vi "Gas_Setup.vi"() -> ()   [LabVIEW 2013]
uses:
  ADAM Controls/Ch_description_ADAM.ctl
  ADAM Controls/Module_type_ADAM.ctl
  ADAM Controls/Function_ADAM.ctl
  ADAM Controls/Channel_State.ctl
  ADAM Controls/Calib_type_ADAM.ctl
  ADAM Controls/Address.ctl
  ADAM Controls/Shut_Off_Valve.ctl
  ADAM Controls/Channel_names.ctl
  ADAM Controls/Update_scan_value.ctl
  Anemometry/Anemometry Sub Vis/Globals/Preference_global.vi
panel:
  out "Ch names":string[](array[string])
  in  "Select Plug Ins":bool
  in  "Source Info":string[][](table)
  in  "Trace Very Low":T1
  in  "Carrier 1 Very Low":T1
  in  "Carrier 1 Hi-Tec Range":u16(ring) items=["Very Low", "Low", "High"]
  in  "Trace Hi-Tec Range":u16(ring) items=["Very Low", "Low", "High"]
  in  "Carrier 1 High":T1
  in  "Carrier 1 Low":T1
  in  "Trace Low":T1
  in  "Trace High":T1
  in  "Release Orientation":u16(ring) items=["Vertical", "Horizontal 0 Deg", "Downwards", "External System Tests", "Horizontal", "Edit Strings"]
  in  "Source Type":u16(ring) items=["11mm downward facing", "1mm Annulus above tank wall with Internal 2mm Annulus floating roof at 50mm.", "23mm IDD=8mm", "2mm Annulus around a quarter of inside of tank wall", "2mm Annulus around inside of tank wall", "4 point source ID=8.5mm located 90 deg apart on 8cm Diameter", "8mm Annulus around inside of tank wall", "B2 D=6.8mm", "B204 Height 244mm ID 5.5mm", "B230 Height 152.4mm ID 8.5mm", "B30 Area", "B311 ID=11mm", "B331 ID=5.4mm", "B38_8mm_ID_passive", "B38_OD=3.1mm_ID=2mm", "B548 OD=13.8mm ID=3.5mm", "D=12mm", "D=13.6mm", "D=16mm (ID=12 mm)", "D=18mm", "D=20mm", "D=22.5mm", "D=3.4mm", "D=5mm (ground release)", "D=6mm (ID=4.2 mm)", "D=7.1mm", "D=9mm", "D=9mm  20mm long passive", "Dext = 8.5 mm", "Exit Port of Solenoid Valve", "H=25:W=100mm", "H=50", "ID=15 mm 90 deg bend copper tube", "ID=5.1mm OD=5.8mm (Ground release)", "ID=5.1mm OD=5.8mm (roof release)", "ID=5mm OD=5.8mm", "ID=8.5mm OD=10mm", "ID=9.5mm OD=12.5mm", "Line Source 100mm  1.07m width", "Line Source 25mm  1.3m long  perp to flow", "Line Source 25x1300", "Line Source 50mm  1.07m Wide", "Line source parallel to flow", "None", "ROSE 9mm at last grid", "SAV ID=3.5mm", "Sample tubes in source", "Single 5mm Stack", "Single 7.9 mm stack", "THORP  ID=5.1mm", "Twin 5mm Stacks", "Twin Passive Stacks ID=8mm OD=8.7mm", "UKAEA ID=1.7mm", "W=50mm", "Edit Strings"]
  in  "Current Release Temp":dbl format="%.2f"
  in  "Release Temperature":u16(ring) items=["Enter Value", "EnFlo_Tunnel:Job:Name", "GMU:Source:Type", "GMU:Release:Orientation", "EnFlo_Tunnel:Obstacle/:Building", "EnFlo_Tunnel:Vorticity:Generators", "EnFlo_Tunnel:Roughness:Height", "EnFlo_Tunnel:Side Wall:Separation", "GMU:Trace:Gas", "GMU:Carrier 1:Gas", "GMU:Carrier 2:Gas", "GMU:Carrier 1:Hi-Tec Range", "GMU:Trace:Hi-Tec Range", "EnFlo_Tunnel:Obstacle:Orientation", "GMU:Source:Density Ratio", "GMU:Carrier 1:Dem Volt", "GMU:Carrier 2:Dem Volt", "GMU:Trace:Dem Volt", "GMU:Carrier 1:Meas Volt", "GMU:Carrier 2:Meas Volt", "GMU:Trace:Meas Volt", "GMU:Carrier 1:Meas Q", "GMU:Carrier 2:Meas Q", "GMU:Trace:Meas Q", "GMU:Carrier 1:Meas M_dot", "GMU:Carrier 2:Meas M_dot", "GMU:Trace:Meas M_dot", "GMU:Remaining:Nitrogen", "GMU:Remaining:Helium", "GMU:Remaining:CO2", "GMU:Remaining:Krypton", "GMU:Remaining:Ethane", "GMU:Remaining:Propane", "GMU:Calibration:Gas 1", "GMU:Calibration:Gas 2", "GMU:Signal FID:Calib Gas", "GMU:Source:Dem Q", "GMU:Source:Meas Q", "GMU:Source:Meas M_dot", "GMU:Source:Meas Density", "GMU:Source:Meas Den Ratio", "GMU:Source:Dem Strength", "GMU:Source:Meas Strength", "GMU:Source:Est Time", "GMU:Detector:Meas Current", "GMU:Detector:Strength", "Froude:NPL:Atmos_Press", "EnFlo Lab:Hygrometry:Rel Humidity", "EnFlo Lab:Hygrometry:Dew Point temp", "EnFlo Lab:Hygrometry:Air Temp", "GMU:Test:Ethane trip", "EnFlo_Tunnel:Safety:GMU_Watchdog", "EnFlo_Tunnel:Speed:Dem Velocity", "EnFlo_Tunnel:Speed:Calib Tweak", "EnFlo_Tunnel:Speed:Dem Current", "EnFlo_Tunnel:Usonic Fixed:Velocity", "EnFlo_Tunnel:Usonic Fixed:Direction", "EnFlo_Tunnel:Prop Y+ve:Velocity", "EnFlo_Tunnel:Prop Y-ve:Velocity", "EnFlo_Tunnel:Shaft:rpm", "EnFlo_Tunnel:Reference:Velocity", "EnFlo_Tunnel:Hydrosonic:Integral", "EnFlo_Tunnel:Days Run at:2.5m/s", "Hydrosonic:Transducer:Setting", "EnFlo_Tunnel:Trav Origin:X Offset", "EnFlo_Tunnel:Trav Pos:X", "EnFlo_Tunnel:Trav Pos:Y", "EnFlo_Tunnel:Trav Pos:Z", "EnFlo Lab:labstrat1:Z=4.5m", "EnFlo Lab:labstrat1:Z=3.5m", "EnFlo Lab:labstrat1:Z=2.5m", "EnFlo Lab:labstrat1:Z=1.5m", "EnFlo Lab:labstrat1:Z=0.5m", "EnFlo Lab:labstrat1:Delta T", "EnFlo Lab:Desired:Air Temp", "EnFlo Lab:Heat:Extraction", "EnFlo Lab:labstrat1:Av Temp", "University:Outside:Temp", "EnFlo_Tunnel:Inlet Heater:Temp 1", "EnFlo_Tunnel:Inlet Heater:Temp 2", "EnFlo_Tunnel:Inlet Heater:Temp 3", "EnFlo_Tunnel:Inlet Heater:Temp 4", "EnFlo_Tunnel:Inlet Heater:Temp 5", "EnFlo_Tunnel:Inlet Heater:Temp 6", "EnFlo_Tunnel:Inlet Heater:Temp 7", "EnFlo_Tunnel:Inlet Heater:Temp 8", "EnFlo_Tunnel:Inlet Heater:Temp 9", "EnFlo_Tunnel:Inlet Heater:Temp 10", "EnFlo_Tunnel:Inlet Heater:Temp 11", "EnFlo_Tunnel:Inlet Heater:Temp 12", "EnFlo_Tunnel:Inlet Heater:Temp 13", "EnFlo_Tunnel:Inlet Heater:Temp 14", "EnFlo_Tunnel:Inlet Heater:Temp 15", "EnFlo_Tunnel:Inlet Heater:Av Temp", "EnFlo_Tunnel:Inlet Heater:Max Temp", "EnFlo_Tunnel:Heater:Enable", "EnFlo_Tunnel:floor near:1", "EnFlo_Tunnel:floor near:3", "EnFlo_Tunnel:floor near:5", "EnFlo_Tunnel:floor far:7", "EnFlo_Tunnel:floor near:7", "EnFlo_Tunnel:floor far:9", "EnFlo_Tunnel:floor near:10", "EnFlo_Tunnel:floor near:11", "EnFlo_Tunnel:floor far:11", "EnFlo_Tunnel:Exit Duct:Temp", "EnFlo_Tunnel:Parker X:Temp", "EnFlo_Tunnel:roof near:19", "EnFlo_Tunnel:roof far:19", "EnFlo_Tunnel:Fan Gearbox:Y+ Temp", "EnFlo_Tunnel:Fan Gearbox:Y- Temp", "B_Tunnel:Motor:Temp", "Uni:Chilled Water:Temp", "EnFlo_Tunnel:Chilled Water:Motor1 Temp", "EnFlo_Tunnel:Chilled Water:Motor2 Temp", "EnFlo_Tunnel:Chilled Water:Supply", "EnFlo_Tunnel:Chilled Water:Return", "EnFlo_Tunnel:Chilled Water:Dem Temp", "EnFlo_Tunnel:Chilled Water:Valve Dem Pos", "EnFlo_Tunnel:Chilled Water:Valve Dem Voltage", "A_Tunnel:Trav:1", "A_Tunnel:Speed:Dem Velocity", "A_Tunnel:Speed:Calib Tweak", "A_Tunnel:Speed:Dem Voltage", "A_Tunnel:Motor:Temp", "GMU:Source:Release Temp", "Complete:Scan:Period", "D_Tunnel:Motor:Temp", "Cluster Room:General:Temp", "Cluster Room:Temp:Warning", "D_Tunnel:Speed:Dem Velocity", "D_Tunnel:Speed:Calib Tweak", "D_Tunnel:Speed:Dem Voltage", "EnFlo Lab:Underfloor Tank:Temp", "Laser:Cooling water:Return Temp", "EnFlo_Tunnel:User:Name", "A_Tunnel:User:Name", "D_Tunnel:User:Name", "Paul_Hayden:User:Name", "Uni:Chilled Water:Temp Warning", "Frauke_Desktop:User:Name", "ADAM_Server:User:Name", "Calibration_Tunnel:User:Name", "EnFlo_Tunnel:Side near:10", "EnFlo_Tunnel:Side far:10", "EnFlo_Tunnel:Source_Pos:X", "EnFlo_Tunnel:Source_Pos:Y", "EnFlo_Tunnel:Source_Pos:Z", "EnFlo_Tunnel:Max_Surface:Temp", "EnFlo_Tunnel:Chiller_Pump:Enable", "A_Tunnel:Motor:Enable", "GMU:Source:Divertor Valve", "EnFlo_Tunnel:Tap_Water:Enable", "EnFlo_Tunnel:Cooling_Panel:Manifold_Temp", "EnFlo_Tunnel:Motor:Enable", "EnFlo_Tunnel:Lights:Enable", "EnFlo_Tunnel:FFID:Temp", "GMU:Gas:Enable", "GMU:Detector:Happy", "EnFlo_Tunnel:Gas Solenoid:Status", "EnFlo_Tunnel:Usonic Inlet Z=75:Velocity", "EnFlo_Tunnel:Usonic Inlet Z=75:Direction", "GMU:Source:Pressure", "EnFlo_Tunnel:Wind:Direction", "Status:of:PB_G4_2", "PB_G4_2:User:Name", "EnFlo Lab:Comp Air:Pressure", "EnFlo Lab:Leak_Detector:Happy", "Paul_Desk:User:Name", "EnFlo Lab:Comp Air:Warning", "EnFlo_Tunnel:Turbine_1:Dem_Volts", "Laser:Cooling_Pump:Enable", "LDA:System:Enable", "FFID:System:Enable", "EnFlo_Tunnel:Motor:Temp", "Laser:Cooling water:Temp Warning", "GMU:Trace:Open", "No Match::", "EnFlo_Tunnel:Chiller_Pump:Running", "EnFlo_Tunnel:Parker X:Warning Temp", "B_Tunnel:User:Name", "EnFlo_Tunnel:Heat_Ex_Water:Return Temp", "EnFlo_Tunnel:Exit Duct Top:Temp", "LDA:3 Phase:Power", "Hydrosonic:Seeder:Enable", "Sugar:Water:Temp", "Hydrosonic:Tank:Temp", "A_Tunnel:Turbine:Enable", "A_Tunnel:Turbine_1:Dem_Volts"]
  in  "Gas Remaining":string[][](table)
  in  "Signal FID Calib Gas":dbl format="%.2f"
  in  "Signal FID Calib Channel":u16(ring) items=["Input Value", "Channel 1", "Channel 2"]
  in  "Channel 2":dbl format="%.2f"
  in  "Channel 1":dbl format="%.2f"
  in  "Carrier 2 Gas":u16(ring) items=["Air", "Nitrogen", "Helium", "CO2", "Krypton", "None"]
  in  "Trace Gas":u16(ring) items=["Propane", "Ethane"]
  in  "Carrier 1 Gas":u16(ring) items=["Air", "Nitrogen", "Helium", "CO2", "Krypton", "None"]
  out "Numerical Values":dbl[](array[numeric]) format="%.9f"
  out "Ch Description Array":T2[](array[typedef]) {"Duty" format="%.0b"; "D" format="%#_5g"; "C" format="%#_5g"; "B" format="%#_5g"; "A" format="%#_5g"}
  out "dup reference":refnum<vi>
  in  "stop":bool
  in  "OK":bool
  # "Calibration Gas (ppm)"
  # "Very\nLow\nRange"
  # "High\nRange"
  # "Low\nRange"
  # "Low\nRange"
  # "Very\nLow\nRange"
  # "High\nRange"
  # "Dispersion Setup"
  # "To Source"
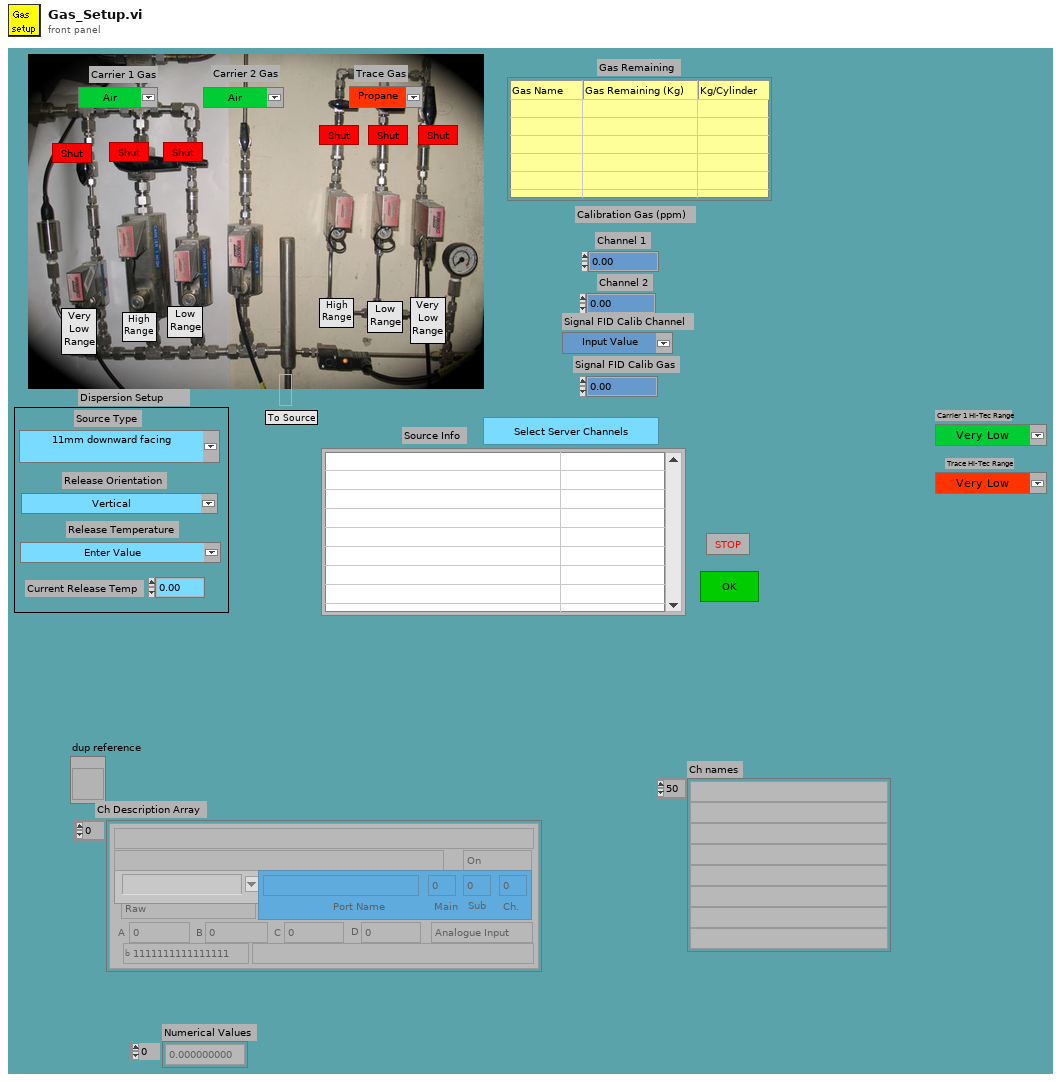
[diagram p1: front panel]
types:
  T1 = typedef "Shut_Off_Valve.ctl" = bool
  T2 = typedef "Ch_description_ADAM.ctl" = cluster{"Ch Name":string, "Type":T3, "Function":T4, "Ch State":T5, "Calibration type":T6, "A":dbl, "B":dbl, "C":dbl, "D":dbl, "Comments":string, "Address":T7, "String":string, "Duty":u16}
  T3 = typedef "Module_type_ADAM.ctl" = string
  T4 = typedef "Function_ADAM.ctl" = enum16{"Analogue Input", "Digital Input", "Event counter", "Event rate", "Analogue Output", "Digital Output", "Relay Output"}
  T5 = typedef "Channel_State.ctl" = enum16{"On", "Off", "Always On", "Always Off"}
  T6 = typedef "Calib_type_ADAM.ctl" = enum16{"Raw", "Bx + A", "Cx^2 + Bx + A", "Dx^3 + Cx^2 + Bx + A", "In Band", "Hi-Tec Q", "Hi-Tec M_dot", "Text"}
  T7 = typedef "Address.ctl" = cluster{"Main":i32, "Ch.":i32, "Sub":i32, "Port Name":string}
  T8 = typedef "Channel_names.ctl" = enum16{"Active Only", "Active + Off", "All Channels"}
  T9 = typedef "Update_scan_value.ctl" = cluster{"Channel Name":string, "New Value":dbl}
  T10 = enum16{"Zero or one", "One", "Zero or more", "One or more"}
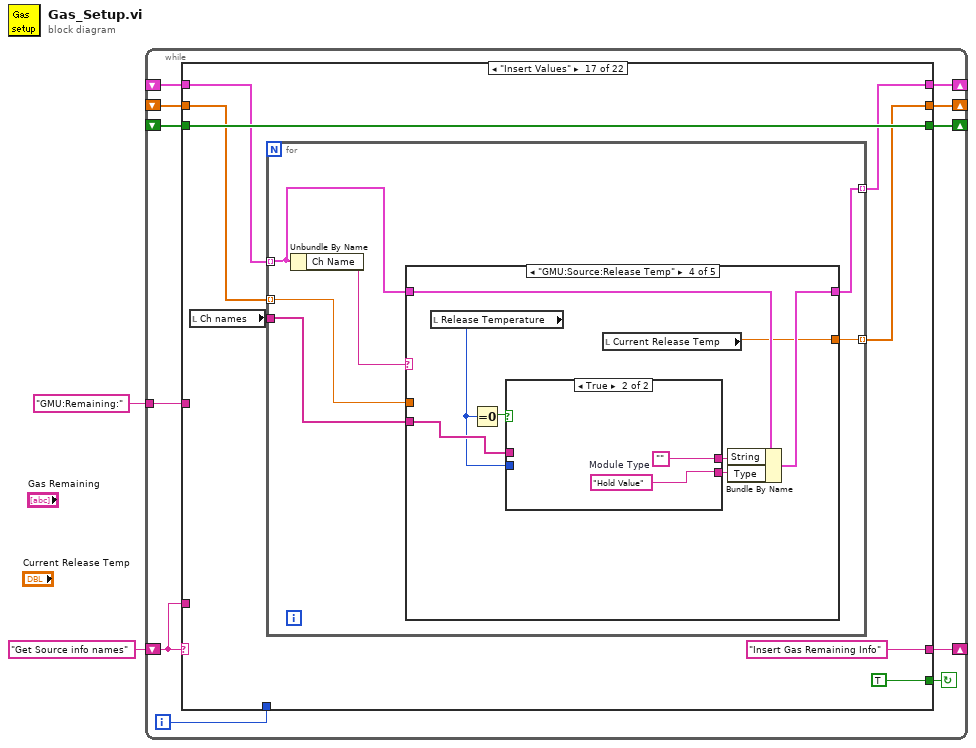
[diagram p0: block diagram]
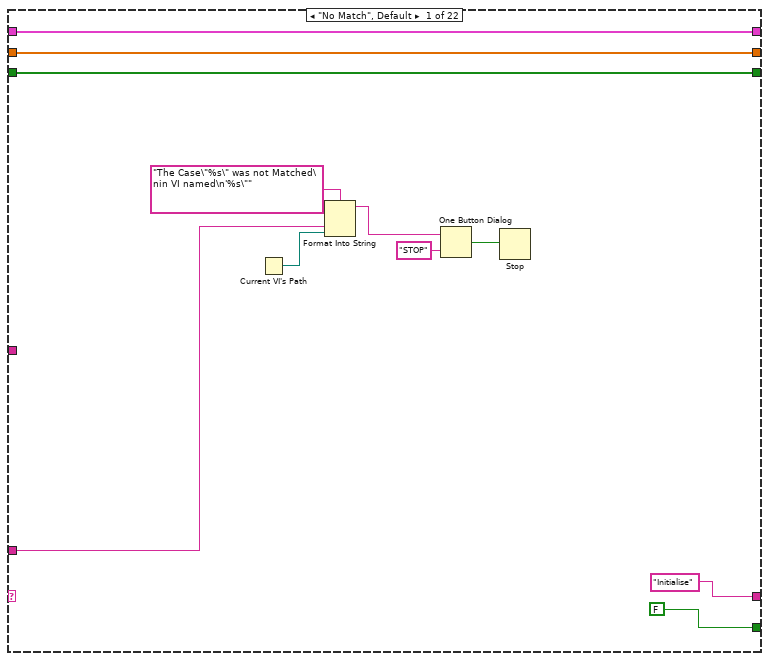
[diagram p2: hidden frame]
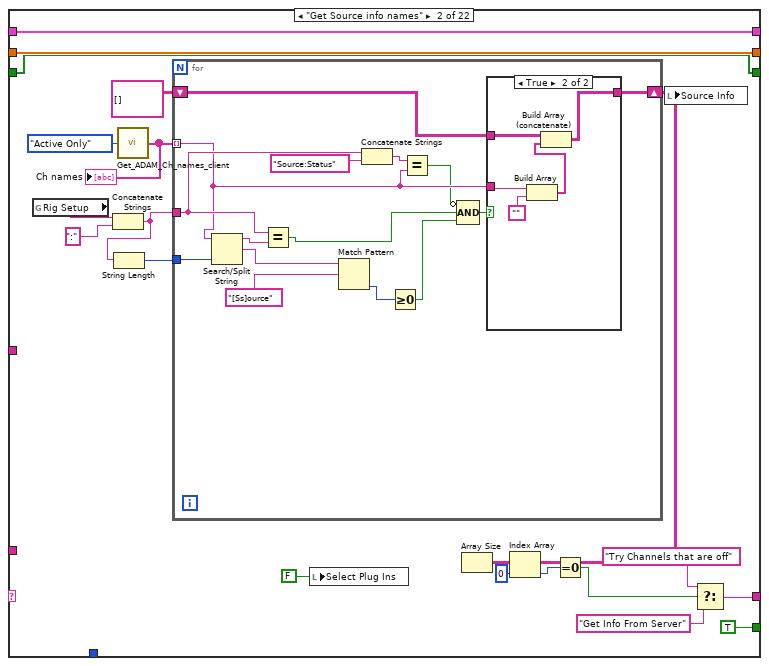
[diagram p3: hidden frame]
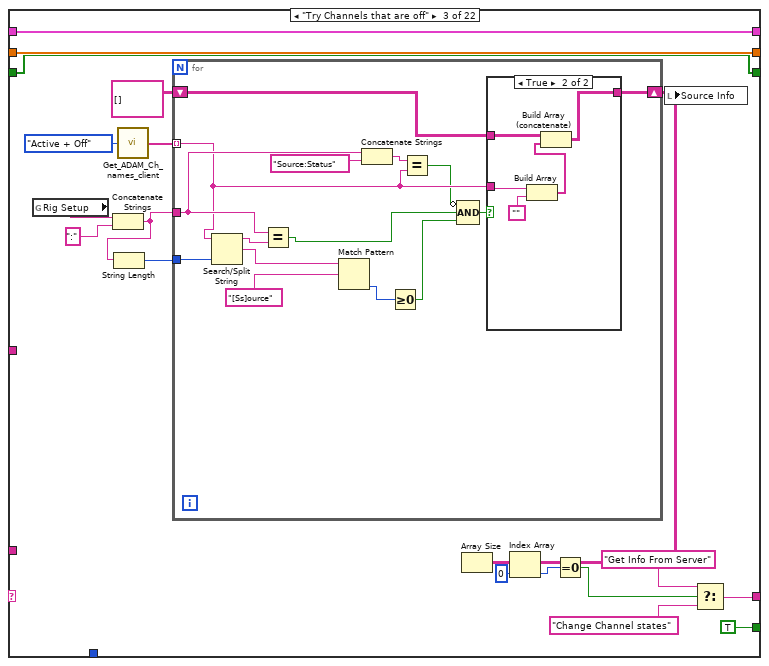
[diagram p5: hidden frame]
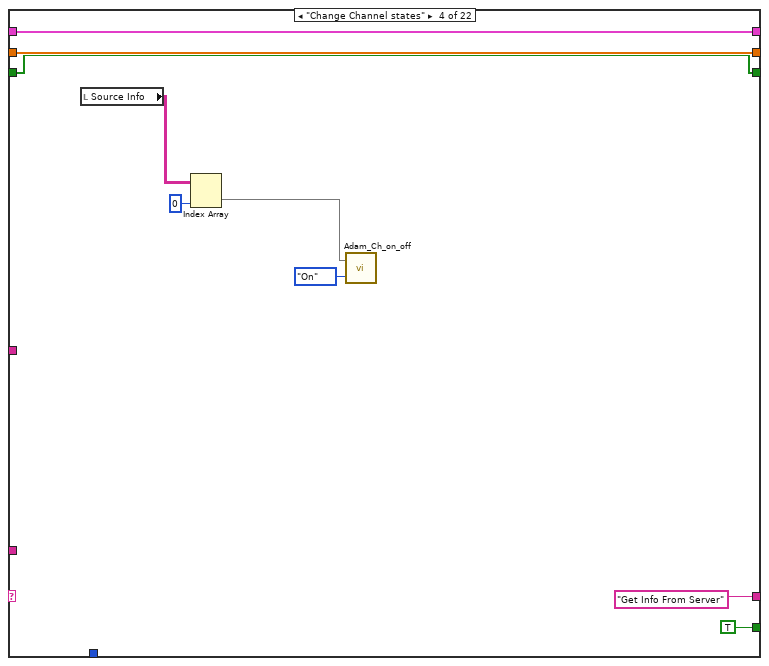
[diagram p7: hidden frame]
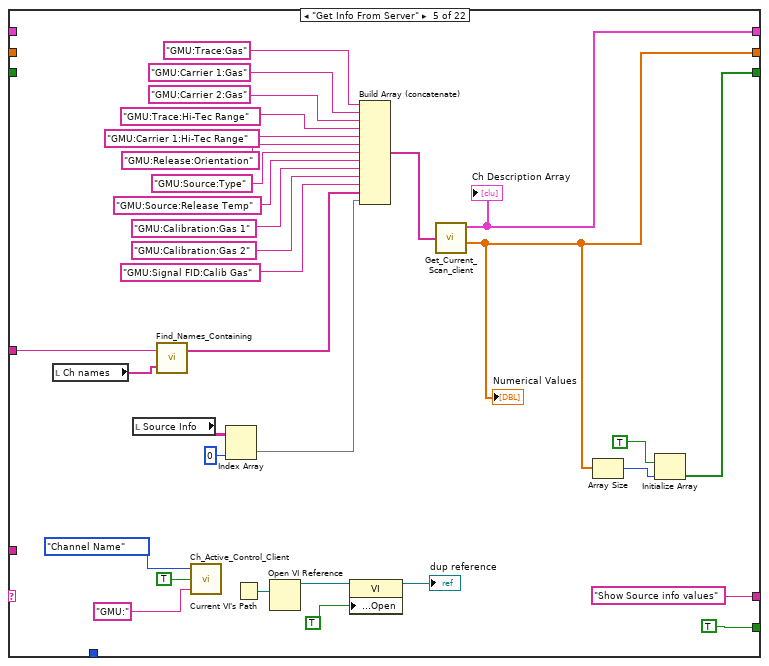
[diagram p8: hidden frame]
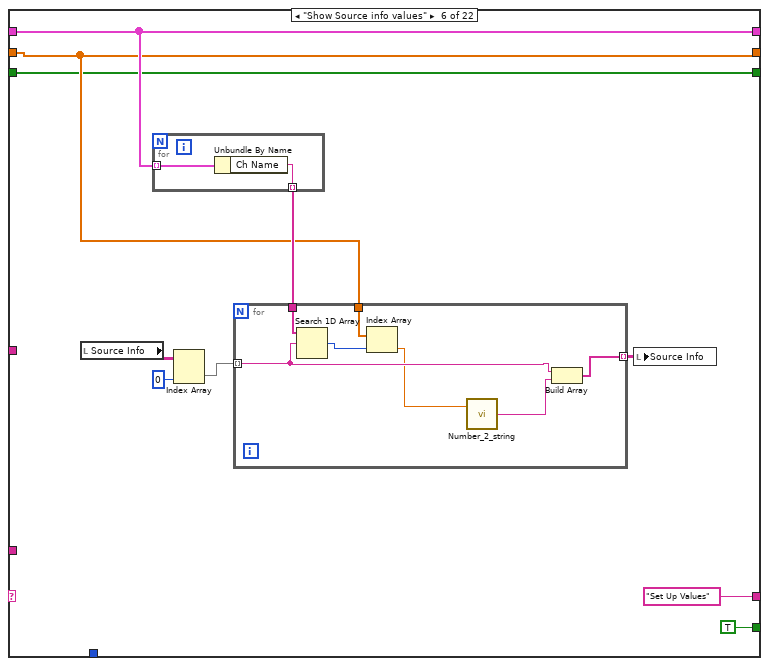
[diagram p9: hidden frame]
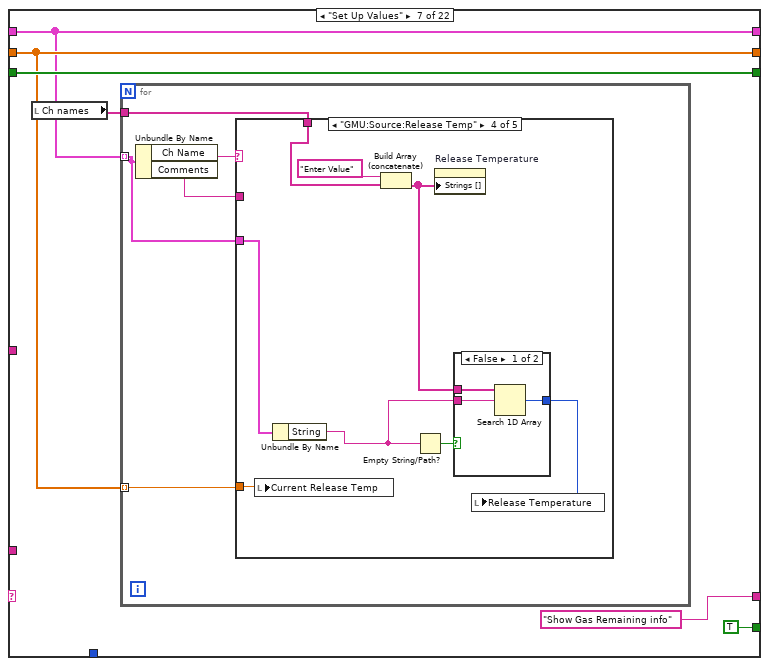
[diagram p10: hidden frame]
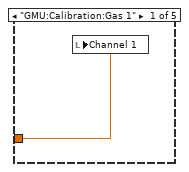
[diagram p11: hidden frame]
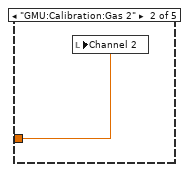
[diagram p12: hidden frame]
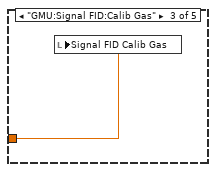
[diagram p13: hidden frame]
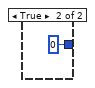
[diagram p14: hidden frame]
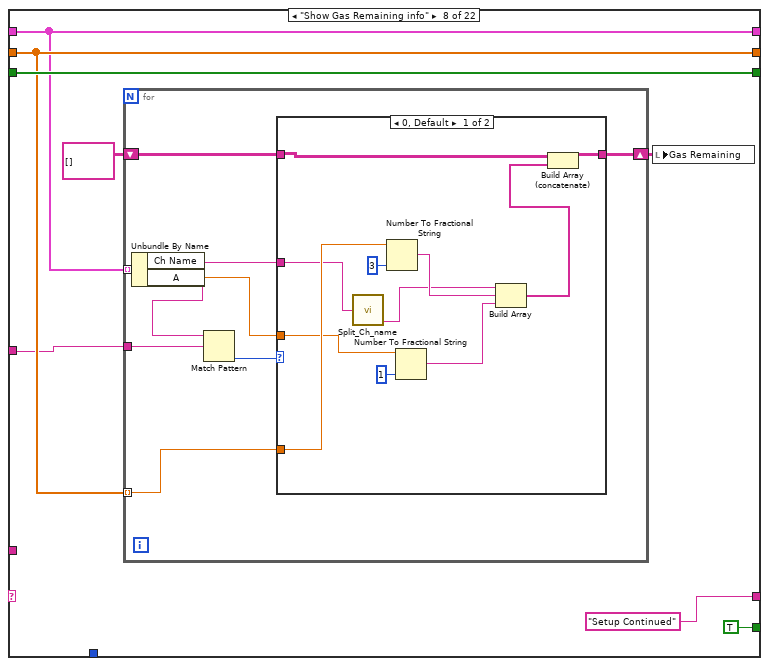
[diagram p16: hidden frame]
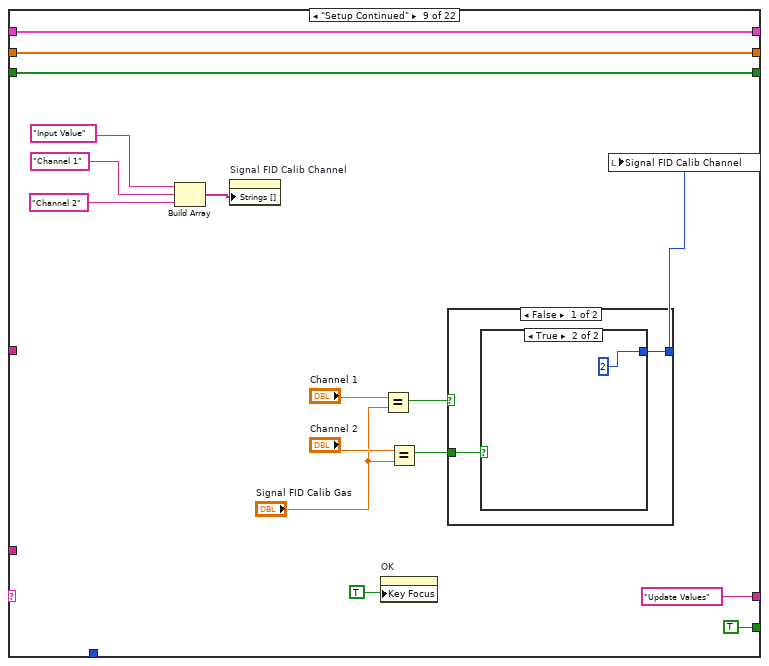
[diagram p18: hidden frame]
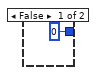
[diagram p19: hidden frame]
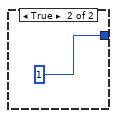
[diagram p20: hidden frame]
diagram:
  n1 = while {
    shift-left: _ -> [w5]
    shift-right: [w6] -> _
    shift-left: _ -> [w7]
    shift-right: [w9] -> _
    shift-left: _ -> [w8]
    shift-right: [w10] -> _
    shift-left: "Get Source info names" ("t") -> [w11]
    shift-right: [w12] -> _
    tunnel: "GMU:Remaining:" -> [w3]
    i -> [w4]
    stop <- w13 continue-if-true
    n2 = case shown="\"Insert Values\"" w11 {
      tunnel: [FALSE TRUE ("T button?") TRUE ("T button?") TRUE ("T button?") TRUE TRUE ("T button?") TRUE ("T button?") TRUE ("T button?") TRUE ("T button?") TRUE ("T button?") TRUE ("T button?") TRUE ("T button?") TRUE ("T button?") TRUE ("T button?") TRUE ("T button?") TRUE ("T button?") TRUE ("T button?") TRUE ("T button?") TRUE ("T button?") TRUE ("T button?") TRUE ("T button?") FALSE ("T button?")] -> w13
      tunnel: ["Initialise" w26 w68 "Get Info From Server" "Show Source info values" "Set Up Values" "Show Gas Remaining info" "Setup Continued" "Update Values" "Slow FID Calib Gas" w324 "Update Release Temperature" "Sort out Valve Logic" "Hi Tec Ranges" "Continue looping?" w468 "Insert Gas Remaining Info" "Insert Source info values" "Update Server" w566 "Get Source info names" ("t") "End"] -> w12
      tunnel: w11 -> [w19 _ _ _ _ _ _ _ _ _ _ _ _ _ _ _ _ _ _ _ _ _]
      tunnel: [w16 w40 w80 w114 w139 w155 w167 w195 w235 w246 w329 w347 w377 w394 w452 w474 w476 w515 w547 w575 w631 w682] -> w10
      tunnel: [w15 w39 w79 w113 w125 w154 w168 w196 w234 w244 w328 w346 w376 w393 w451 w473 w479 w521 w549 w574 w630 w681] -> w9
      tunnel: w8 -> [w16 w40 w80 w114 _ w155 w167 w195 w235 w247 w329 w347 w377 w394 w452 w474 w477 w515 w547 w575 w631 w682]
      tunnel: w7 -> [w15 w39 w79 w113 _ w154 w168 w196 w234 w245 w328 w346 w376 w393 w451 w473 w478 w520 w550 w574 w630 w681]
      tunnel: [w14 w38 w78 w112 w124 w153 w170 w198 w232 w241 w322 w344 w374 w391 w449 w467 w481 w523 w546 w573 w629 w674] -> w6
      tunnel: w5 -> [w14 w38 w78 w112 _ w153 w170 w198 w232 w242 w322 w344 w374 w391 w449 w467 w481 w523 w546 w573 w629 w674]
      tunnel: w4 -> [_ _ _ _ _ _ _ _ _ _ w321 _ _ _ _ _ _ _ _ _ _ _]
      tunnel: w3 -> [_ _ _ _ w122 _ _ w194 _ _ _ _ _ _ _ _ _ w514 _ _ _ _]
      frame "No Match", Default {
        n3 = Current VI's Path() -> (path=w18:path)
        n4 = Format Into String(format string="The Case\"%s\" was not Matched\nin VI named\n'%s\"" ("Format String"), w19, w18) -> (resulting string=w22:string)  [unwired: 2 in, 1 out]
        n5 = One Button Dialog(message=w22, button name ("OK")="STOP") -> (true=w20:bool)
        n6 = Stop(stop? (T)=w20) -> ()
      }
      frame "Get Source info names" {
        n7 = global read "Preference_global.vi" "Rig Setup"() -> (w44:string)
        n8 = Concatenate Strings(w44, ":" ("string")) -> (w41:string)
        n9 = String Length(string=w41) -> (length=w42:i32)
        n10 = call "Get_ADAM_Ch_names_client.vi"("Channel names set"=Channel_names."Active Only") -> ("Ch names"=w35:string[])
        "Ch names" <- w35
        n11 = for {
          tunnel: w42 -> [w59]
          tunnel: w35 -> [w49] mode=indexing
          tunnel: w41 -> [w51]
          shift-right: [w53] -> w33
          shift-left: string[][] [] -> [w54]
          n12 = Search/Split String(string=w49, offset (0)=w59) -> (substring before match=w58:string, match + rest of string=w57:string)  [unwired: 2 out]
          n13 = Equal?(x=w51, y=w58) -> (x = y?=w47:bool)
          n14 = Match Pattern(string=w57, regular expression="[Ss]ource") -> (offset past match=w55:i32)  [unwired: 4 out]
          n15 = Concatenate Strings(w51, "Source:Status") -> (w50:string)
          n16 = Greater Or Equal To 0?(x=w55) -> (x >= 0?=w48:bool)
          n17 = Equal?(x=w50, y=w49) -> (x = y?=w46:bool)
          n18 = Compound Arithmetic op=AND(invert w46, w47, w48) -> (w45:bool)
          n19 = case shown="True" w45 {
            tunnel: w54 -> [w60 w65]
            tunnel: w49 -> [_ w63]
            tunnel: [w60 w64] -> w53
            frame False {
            }
            frame True {
              n20 = Build Array(w63, "") -> (w61:string[])
              n21 = Build Array (concatenate)(w65, w61) -> (w64:string[][])
            }
          }
        }
        n22 = local write "Select Plug Ins"(FALSE ("Select Plug Ins")) -> ()
        n23 = Array Size(array=w33) -> (size(s)=w32:i32[])
        n24 = Index Array(array=w32, index=0) -> (element=w30:i32)
        n25 = Equal To 0?(x=w30) -> (x = 0?=w28:bool)
        n26 = local write "Source Info"(w33) -> ()
        n27 = Select(t="Try Channels that are off", s=w28, f="Get Info From Server") -> (s? t:f=w26:string)
      }
      frame "Try Channels that are off" {
        n28 = global read "Preference_global.vi" "Rig Setup"() -> (w84:string)
        n29 = Concatenate Strings(w84, ":" ("string")) -> (w81:string)
        n30 = String Length(string=w81) -> (length=w82:i32)
        n31 = call "Get_ADAM_Ch_names_client.vi"("Channel names set"=Channel_names."Active + Off") -> ("Ch names"=w75:string[])
        n32 = for {
          tunnel: w82 -> [w99]
          tunnel: w75 -> [w89] mode=indexing
          tunnel: w81 -> [w91]
          shift-right: [w93] -> w74
          shift-left: string[][] [] -> [w94]
          n33 = Search/Split String(string=w89, offset (0)=w99) -> (substring before match=w98:string, match + rest of string=w97:string)  [unwired: 2 out]
          n34 = Equal?(x=w91, y=w98) -> (x = y?=w87:bool)
          n35 = Match Pattern(string=w97, regular expression="[Ss]ource") -> (offset past match=w95:i32)  [unwired: 4 out]
          n36 = Concatenate Strings(w91, "Source:Status") -> (w90:string)
          n37 = Greater Or Equal To 0?(x=w95) -> (x >= 0?=w88:bool)
          n38 = Equal?(x=w90, y=w89) -> (x = y?=w86:bool)
          n39 = Compound Arithmetic op=AND(invert w86, w87, w88) -> (w85:bool)
          n40 = case shown="True" w85 {
            tunnel: w94 -> [w100 w105]
            tunnel: w89 -> [_ w103]
            tunnel: [w100 w104] -> w93
            frame False {
            }
            frame True {
              n41 = Build Array(w103, "") -> (w101:string[])
              n42 = Build Array (concatenate)(w105, w101) -> (w104:string[][])
            }
          }
        }
        n43 = Array Size(array=w74) -> (size(s)=w73:i32[])
        n44 = Index Array(array=w73, index=0) -> (element=w71:i32)
        n45 = Equal To 0?(x=w71) -> (x = 0?=w69:bool)
        n46 = local write "Source Info"(w74) -> ()
        n47 = Select(t="Get Info From Server", s=w69, f="Change Channel states") -> (s? t:f=w68:string)
      }
      frame "Change Channel states" {
        n48 = local read "Source Info"() -> (w109:string[][])
        n49 = Index Array(array=w109, index (col)=0 ("disabled index (col)")) -> (element=w107:string[])  [unwired: 1 in]
        n50 = call "Adam_Ch_on_off.vi"("Ch State"=Channel_State."On", "ADAM Ch Names"=w107) -> ()  [unwired: 1 out]
      }
      frame "Get Info From Server" {
        n51 = local read "Ch names"() -> (w115:string[])
        n52 = local read "Source Info"() -> (w118:string[][])
        n53 = call "Find_Names_Containing.vi"("Ch names"=w115, "String to match"=w122) -> ("Matched Names"=w123:string[])  [unwired: 1 out]
        n54 = call "Ch_Active_Control_Client.vi"("Match"="GMU:", "Activate Channels?"=TRUE, "Control on"=enum16{"Channel Name", "Main Address"}."Channel Name") -> ()  [unwired: 2 out]
        n55 = Index Array(array=w118, index (col)=0 ("disabled index (col)")) -> (element=w116:string[])  [unwired: 1 in]
        n56 = Current VI's Path() -> (path=w141:path)
        n57 = Open VI Reference(vi path=w141) -> (vi reference=w142:refnum<vi>)  [unwired: 1 in, 5 out]
        n58 = property class="VI"(reference=w142, "Front Panel Window:Open"=TRUE) -> (reference out=→"dup reference":refnum<vi>)  [unwired: 1 in, 1 out]
        n59 = Build Array (concatenate)("GMU:Trace:Gas", "GMU:Carrier 1:Gas", "GMU:Carrier 2:Gas", "GMU:Trace:Hi-Tec Range", "GMU:Carrier 1:Hi-Tec Range", "GMU:Release:Orientation", "GMU:Source:Type", "GMU:Source:Release Temp", "GMU:Calibration:Gas 1", "GMU:Calibration:Gas 2", "GMU:Signal FID:Calib Gas", w123, w116) -> (w144:string[])
        n60 = call "Get_Current_Scan_client.vi"("ADAM Ch Names"=w144) -> ("Ch Description Array"=w139:T2[], "Numerical Values"=w125:dbl[])  [unwired: 2 out]
        "Ch Description Array" <- w139
        "Numerical Values" <- w125
        n61 = Array Size(array=w125) -> (size(s)=w127:i32)
        n62 = Initialize Array(TRUE, w127) -> (w124:bool[])
      }
      frame "Show Source info values" {
        n63 = local read "Source Info"() -> (w149:string[][])
        n64 = for {
          tunnel: w155 -> [w165] mode=indexing
          tunnel: [w164] -> w156 mode=indexing
          n65 = Unbundle By Name(w165) -> ("Ch Name"=w164:string)
        }
        n66 = Index Array(array=w149, index (col)=0 ("disabled index (col)")) -> (element=w147:string[])  [unwired: 1 in]
        n67 = for {
          tunnel: w156 -> [w163]
          tunnel: w147 -> [w160] mode=indexing
          tunnel: w154 -> [w161]
          tunnel: [w157] -> w152 mode=indexing
          n68 = Search 1D Array(1D array=w163, element=w160) -> (index of element=w162:i32)  [unwired: 1 out]
          n69 = Index Array(array=w161, index=w162) -> (element=w159:dbl)
          n70 = call "Number_2_string.vi"("number"=w159) -> ("String"=w158:string)  [unwired: 1 in]
          n71 = Build Array(w160, w158) -> (w157:string[])
        }
        n72 = local write "Source Info"(w152) -> ()
      }
      frame "Set Up Values" {
        n73 = local read "Ch names"() -> (w166:string[])
        n74 = for {
          tunnel: w168 -> [w172] mode=indexing
          tunnel: w167 -> [w174] mode=indexing
          tunnel: w166 -> [w173]
          n75 = Unbundle By Name(w174) -> ("Ch Name"=w176:string, "Comments"=w175:string)
          n76 = case shown="\"GMU:Source:Release Temp\"" w176 {
            tunnel: w172 -> [w177 w178 w179 w183 _]
            tunnel: w175 -> [_ _ _ _ _]
            tunnel: w174 -> [_ _ _ w187 _]
            tunnel: w173 -> [_ _ _ w181 _]
            frame "GMU:Calibration:Gas 1" {
              n77 = local write "Channel 1"(w177) -> ()
            }
            frame "GMU:Calibration:Gas 2" {
              n78 = local write "Channel 2"(w178) -> ()
            }
            frame "GMU:Signal FID:Calib Gas" {
              n79 = local write "Signal FID Calib Gas"(w179) -> ()
            }
            frame "GMU:Source:Release Temp" {
              n80 = local write "Current Release Temp"(w183) -> ()
              n81 = Unbundle By Name(w187) -> ("String"=w185:string)
              n82 = Build Array (concatenate)("Enter Value", w181) -> (w180:string[])
              n83 = Empty String/Path?(string/path=w185) -> (empty?=w186:bool)
              n84 = property on="Release Temperature" class="Ring (strict)"("Strings []"=w180) -> ()  [unwired: 2 in, 2 out]
              n85 = case shown="False" w186 {
                tunnel: w180 -> [w190 _]
                tunnel: w185 -> [w189 _]
                tunnel: [w188 0 ("index of element")] -> w184
                frame False {
                  n86 = Search 1D Array(1D array=w190, element=w189) -> (index of element=w188:i32)  [unwired: 1 out]
                }
                frame True {
                }
              }
              n87 = local write "Release Temperature"(w184) -> ()
            }
            frame "No Match", Default {
            }
          }
        }
      }
      frame "Show Gas Remaining info" {
        n88 = for {
          tunnel: w196 -> [w202] mode=indexing
          tunnel: w195 -> [w207] mode=indexing
          tunnel: w194 -> [w206]
          shift-right: [w203] -> w192
          shift-left: string[][] [] -> [w204]
          n89 = Unbundle By Name(w207) -> ("Ch Name"=w200:string, "A"=w201:dbl)
          n90 = Match Pattern(string=w200, regular expression=w206) -> (offset past match=w205:i32)  [unwired: 4 out]
          n91 = case shown="0, Default" w205 {
            tunnel: w204 -> [w209 w219]
            tunnel: [w208 w219] -> w203
            tunnel: w202 -> [w213 _]
            tunnel: w201 -> [w212 _]
            tunnel: w200 -> [w211 _]
            frame 0, Default {
              n92 = call "Split_Ch_name.vi"("Ch name"=w211) -> ("Low level"=w215:string)  [unwired: 2 out]
              n93 = Number To Fractional String(number=w213, precision (6)=i16 3) -> (F-format string=w218:string)  [unwired: 2 out]
              n94 = Number To Fractional String(number=w212, precision (6)=i16 1) -> (F-format string=w216:string)  [unwired: 2 out]
              n95 = Build Array(w215, w218, w216) -> (w210:string[])
              n96 = Build Array (concatenate)(w209, w210) -> (w208:string[][])
            }
            frame -1 {
            }
          }
        }
        n97 = local write "Gas Remaining"(w192) -> ()
      }
      frame "Setup Continued" {
        n98 = Build Array("Input Value", "Channel 1", "Channel 2") -> (w226:string[])
        n99 = property on="Signal FID Calib Channel" class="Ring (strict)"("Strings []"=w226) -> ()  [unwired: 2 in, 2 out]
        n100 = property on="OK" class="Bool"("Key Focus"=TRUE ("Write Attribute")) -> ()  [unwired: 2 in, 2 out]
        n101 = Equal?(x="Channel 1", y="Signal FID Calib Gas") -> (x = y?=w225:bool)
        n102 = Equal?(x="Channel 2", y="Signal FID Calib Gas") -> (x = y?=w224:bool)
        n103 = case shown="False" w225 {
          tunnel: [w236 1] -> w220
          tunnel: w224 -> [w237 _]
          frame False {
            n104 = case shown="True" w237 {
              tunnel: [0 2] -> w236
              frame False {
              }
              frame True {
              }
            }
          }
          frame True {
          }
        }
        n105 = local write "Signal FID Calib Channel"(w220) -> ()
      }
      frame "Update Values" {
        n106 = for {
          tunnel: w247 -> [w254] mode=indexing
          tunnel: [w253] -> w246 mode=indexing
          tunnel: w245 -> [w252] mode=indexing
          tunnel: [w251] -> w244 mode=indexing
          tunnel: w242 -> [w250] mode=indexing
          tunnel: [w249] -> w241 mode=indexing
          n107 = Unbundle By Name(w254) -> ("Calibration type"=w257:T6, "String"=w256:string, "Ch Name"=w255:string)
          n108 = case shown="\"Text\"" w257 {
            tunnel: w256 -> [_ w278]
            tunnel: w255 -> [_ w268]
            tunnel: w254 -> [w260 w272]
            tunnel: [w260 w271] -> w253
            tunnel: w252 -> [w259 w270]
            tunnel: [w259 w269] -> w251
            tunnel: w250 -> [w258 w267]
            tunnel: [w258 w261] -> w249
            frame "Raw", Default {
            }
            frame "Text" {
              n109 = call "Get_array_values_fr_String.vi"("String Value"=w278) -> ("String array"=w265:string[])  [unwired: 1 out]
              n110 = To Unsigned Word Integer(number=w270) -> (unsigned 16bit integer=w276:u16)
              n111 = Build Array (concatenate)(w265, "Edit Strings") -> (w264:string[])
              n112 = Array Size(array=w265) -> (size(s)=w277:i32)
              n113 = case shown="\"GMU:Carrier 1:Hi-Tec Range\"" w268 {
                tunnel: [w285 w289 w294 w299 w303 w307 w312 w317] -> w262
                tunnel: w265 -> [_ w287 w291 w297 _ _ _ _]
                tunnel: w276 -> [w285 w290 w295 w300 w304 w308 w313 w318]
                tunnel: w267 -> [_ w288 w293 w298 w302 w306 w311 w316]
                tunnel: w264 -> [_ _ _ _ _ _ w310 w315]
                frame "No match", Default {
                }
                frame "GMU:Trace:Gas" {
                  n114 = property on="Trace Gas" class="Ring (strict)"("Strings []"=w287) -> ()  [unwired: 2 in, 2 out]
                  n115 = Select(t=w290, s=w288, f="Trace Gas") -> (s? t:f=w289:u16)
                  n116 = local write "Trace Gas"(w289) -> ()
                }
                frame "GMU:Carrier 1:Gas" {
                  n117 = property on="Carrier 1 Gas" class="Ring (strict)"("Strings []"=w291) -> ()  [unwired: 2 in, 2 out]
                  n118 = Select(t=w295, s=w293, f="Carrier 1 Gas") -> (s? t:f=w294:u16)
                  n119 = local write "Carrier 1 Gas"(w294) -> ()
                }
                frame "GMU:Carrier 2:Gas" {
                  n120 = property on="Carrier 2 Gas" class="Ring (strict)"("Strings []"=w297) -> ()  [unwired: 2 in, 2 out]
                  n121 = Select(t=w300, s=w298, f="Carrier 2 Gas") -> (s? t:f=w299:u16)
                  n122 = local write "Carrier 2 Gas"(w299) -> ()
                }
                frame "GMU:Carrier 1:Hi-Tec Range" {
                  n123 = Select(t=w304, s=w302, f="Carrier 1 Hi-Tec Range") -> (s? t:f=w303:u16)
                  n124 = local write "Carrier 1 Hi-Tec Range"(w303) -> ()
                }
                frame "GMU:Trace:Hi-Tec Range" {
                  n125 = Select(t=w308, s=w306, f="Trace Hi-Tec Range") -> (s? t:f=w307:u16)
                  n126 = local write "Trace Hi-Tec Range"(w307) -> ()
                }
                frame "GMU:Source:Type" {
                  n127 = property on="Source Type" class="Ring (strict)"("Strings []"=w310) -> ()  [unwired: 2 in, 2 out]
                  n128 = Select(t=w313, s=w311, f="Source Type") -> (s? t:f=w312:u16)
                  n129 = local write "Source Type"(w312) -> ()
                }
                frame "GMU:Release:Orientation" {
                  n130 = property on="Release Orientation" class="Ring (strict)"("Strings []"=w315) -> ()  [unwired: 2 in, 2 out]
                  n131 = Select(t=w318, s=w316, f="Release Orientation") -> (s? t:f=w317:u16)
                  n132 = local write "Release Orientation"(w317) -> ()
                }
              }
              n133 = To Unsigned Word Integer(number=w277) -> (unsigned 16bit integer=w275:u16)
              n134 = Equal?(x=w275, y=w262) -> (x = y?=w261:bool)
              n135 = case shown="True" w261 {
                tunnel: w265 -> [w280 w284]
                tunnel: w268 -> [_ w283]
                tunnel: [w280 w282] -> w273
                tunnel: [w279 w281] -> w263
                tunnel: w262 -> [w279 _]
                frame False {
                }
                frame True {
                  n136 = call "Edit_String_Options_list.vi"("Channel Name"=w283, "String array"=w284) -> ("New Selection Index"=w281:i32, "String array Out"=w282:string[])
                }
              }
              n137 = call "Put_Array_into_String.vi"("String array"=w273) -> ("String Value"=w274:string)
              n138 = Bundle By Name(cluster=w272, "String"=w274) -> (w271:T2)
              n139 = To Double Precision Float(number=w263) -> (double precision float=w269:dbl)
            }
          }
        }
      }
      frame "Slow FID Calib Gas" {
        n140 = Less?(x=w321, y=10) -> (x < y?=w319:bool)
        n141 = case shown="1, Default" "Signal FID Calib Channel" {
          tunnel: "Signal FID Calib Channel" -> [_ w331]
          frame 0 {
          }
          frame 1, Default {
            n142 = case shown="2" w331 {
              tunnel: [0.0 w333 w334] -> w330
              frame 0, Default {
              }
              frame 1 {
                n143 = local read "Channel 1"() -> (w333:dbl)
              }
              frame 2 {
                n144 = local read "Channel 2"() -> (w334:dbl)
              }
            }
            n145 = local write "Signal FID Calib Gas"(w330) -> ()
          }
        }
        n146 = Select(t="Initialise Hi tec selection", s=w319, f="Update Release Temperature") -> (s? t:f=w324:string)
      }
      frame "Initialise Hi tec selection" {
        n147 = local read "Carrier 1 Hi-Tec Range"() -> (w342:u16)
        n148 = local read "Trace Hi-Tec Range"() -> (w338:u16)
        n149 = case shown="2" w342 {
          tunnel: [FALSE FALSE TRUE] -> w341
          tunnel: [FALSE TRUE FALSE] -> w340
          tunnel: [TRUE FALSE FALSE] -> w339
          frame 0, Default {
          }
          frame 1 {
          }
          frame 2 {
          }
        }
        n150 = case shown="0, Default" w338 {
          tunnel: [FALSE FALSE TRUE] -> w335
          tunnel: [FALSE TRUE FALSE] -> w336
          tunnel: [TRUE FALSE FALSE] -> w337
          frame 0, Default {
          }
          frame 1 {
          }
          frame 2 {
          }
        }
        n151 = local write "Carrier 1 Very Low"(w339) -> ()
        n152 = local write "Carrier 1 High"(w341) -> ()
        n153 = local write "Carrier 1 Low"(w340) -> ()
        n154 = local write "Trace Very Low"(w337) -> ()
        n155 = local write "Trace Low"(w336) -> ()
        n156 = local write "Trace High"(w335) -> ()
      }
      frame "Update Release Temperature" {
        n157 = while {
          tunnel: [w380] -> w371
          shift-left: _ -> [w380]
          shift-right: [w381] -> w372
          stop <- FALSE continue-if-true
          n158 = Get Date/Time In Seconds() -> (seconds since 1Jan1904=w378:timestamp)
          n159 = To Double Precision Float(number=w378) -> (double precision float=w381:dbl)
        }
        n160 = local read "Ch names"() -> (w366:string[])
        n161 = Not Equal To 0?(x="Release Temperature") -> (x != 0?=w369:bool)
        n162 = Not Equal?(x=w371, y=w372) -> (x != y?=w370:bool)
        n163 = And(x=w369, y=w370) -> (x .and. y?=w368:bool)
        n164 = case shown="True" w368 {
          tunnel: w366 -> [_ w384]
          tunnel: "Release Temperature" -> [_ w383]
          frame False {
          }
          frame True {
            n165 = Decrement(x=w383) -> (x-1=w382:u16)
            n166 = Index Array(array=w384, index=w382) -> (element=w389:string)
            n167 = Build Array(w389) -> (w388:string[])
            n168 = call "Get_Current_Scan_client.vi"("ADAM Ch Names"=w388) -> ("Numerical Values"=w386:dbl[])  [unwired: 3 out]
            n169 = Index Array(array=w386, index=0) -> (element=w385:dbl)
            n170 = local write "Current Release Temp"(w385) -> ()
          }
        }
      }
      frame "Sort out Valve Logic" {
        n171 = while {
          shift-left: _ -> [w397]
          shift-right: [w396] -> _
          shift-left: _ -> [w398]
          shift-right: [w399] -> _
          shift-left: _ -> [w400]
          shift-right: [w403] -> _
          shift-left: _ -> [w401]
          shift-right: [w402] -> _
          shift-left: _ -> [w404]
          shift-right: [w406] -> _
          shift-left: _ -> [w405]
          shift-right: [w407] -> _
          stop <- FALSE continue-if-true
          n172 = stacked-sequence {
            tunnel: ["Carrier 1 High" _] -> w407
            tunnel: ["Carrier 1 Low" _] -> w406
            tunnel: w405 -> [w416 _]
            tunnel: w404 -> [w415 _]
            tunnel: [_ "Trace Low"] -> w403
            tunnel: [_ "Trace High"] -> w402
            tunnel: w401 -> [_ w430]
            tunnel: w400 -> [_ w429]
            tunnel: ["Carrier 1 Very Low" _] -> w399
            tunnel: w398 -> [w410 _]
            tunnel: w397 -> [_ w431]
            tunnel: [_ "Trace Very Low"] -> w396
            frame #0 {
              n173 = Build Array("Carrier 1 Very Low", "Carrier 1 High", "Carrier 1 Low") -> (w414:T1[])
              n174 = Boolean To (0,1)(Boolean=w414) -> (0, 1=w413:i16[])
              n175 = Add Array Elements(numeric array=w413) -> (sum=w412:i16)
              n176 = case shown="2, Default" w412 {
                tunnel: w416 -> [_ _ w423]
                tunnel: w415 -> [_ _ w422]
                tunnel: "Carrier 1 Very Low" -> [_ _ w425]
                tunnel: w410 -> [_ _ w424]
                tunnel: "Carrier 1 Low" -> [_ _ w421]
                tunnel: "Carrier 1 High" -> [_ _ w420]
                frame 0 {
                }
                frame 1 {
                }
                frame 2, Default {
                  n177 = Exclusive Or(1:w424, 2:w425) -> (0:w419:T1)
                  n178 = Exclusive Or(1:w422, 2:w421) -> (0:w417:T1)
                  n179 = Exclusive Or(1:w423, 2:w420) -> (0:w418:T1)
                  n180 = local write "Carrier 1 Very Low"(w419) -> ()
                  n181 = local write "Carrier 1 High"(w418) -> ()
                  n182 = local write "Carrier 1 Low"(w417) -> ()
                }
              }
            }
            frame #1 {
              n183 = Build Array("Trace Very Low", "Trace High", "Trace Low") -> (w434:T1[])
              n184 = Boolean To (0,1)(Boolean=w434) -> (0, 1=w433:i16[])
              n185 = Add Array Elements(numeric array=w433) -> (sum=w432:i16)
              n186 = case shown="2, Default" w432 {
                tunnel: w430 -> [_ _ w441]
                tunnel: w429 -> [_ _ w440]
                tunnel: "Trace Very Low" -> [_ _ w443]
                tunnel: w431 -> [_ _ w442]
                tunnel: "Trace Low" -> [_ _ w439]
                tunnel: "Trace High" -> [_ _ w438]
                frame 0 {
                }
                frame 1 {
                }
                frame 2, Default {
                  n187 = Exclusive Or(1:w442, 2:w443) -> (0:w437:T1)
                  n188 = Exclusive Or(1:w440, 2:w439) -> (0:w435:T1)
                  n189 = Exclusive Or(1:w441, 2:w438) -> (0:w436:T1)
                  n190 = local write "Trace Very Low"(w437) -> ()
                  n191 = local write "Trace High"(w436) -> ()
                  n192 = local write "Trace Low"(w435) -> ()
                }
              }
            }
          }
        }
      }
      frame "Hi Tec Ranges" {
        n193 = local read "Carrier 1 Very Low"() -> (w445:T1)
        n194 = local read "Trace Very Low"() -> (w446:T1)
        n195 = case shown="True" w445 {
          tunnel: [w455 u16 0 ("Carrier 1 Hi-Tec Range")] -> w444
          frame False {
            n196 = local read "Carrier 1 Low"() -> (w456:T1)
            n197 = Select(t=u16 1 ("Carrier 1 Hi-Tec Range"), s=w456, f=u16 2 ("Carrier 1 Hi-Tec Range")) -> (s? t:f=w455:u16)
          }
          frame True {
          }
        }
        n198 = case shown="False" w446 {
          tunnel: [w460 u16 0 ("Carrier 1 Hi-Tec Range")] -> w447
          frame False {
            n199 = local read "Trace Low"() -> (w461:T1)
            n200 = Select(t=u16 1 ("Carrier 1 Hi-Tec Range"), s=w461, f=u16 2 ("Carrier 1 Hi-Tec Range")) -> (s? t:f=w460:u16)
          }
          frame True {
          }
        }
        n201 = local write "Carrier 1 Hi-Tec Range"(w444) -> ()
        n202 = local write "Trace Hi-Tec Range"(w447) -> ()
      }
      frame "Continue looping?" {
        n203 = local read "Select Plug Ins"() -> (w464:bool)
        n204 = Compound Arithmetic op=OR("stop", "OK", w464) -> (w463:bool)
        n205 = Current VI's Path() -> (path=w471:path)
        n206 = call "Close_Panel_and_Abort.vi"("Vi path"=w471, "stop"="stop") -> ()  [unwired: 1 out]
        n207 = Select(t="Insert Values", s=w463, f="Update Values") -> (s? t:f=w468:string)
      }
      frame "Insert Values" {
        n208 = local read "Ch names"() -> (w475:string[])
        n209 = for {
          tunnel: w477 -> [w485] mode=indexing
          tunnel: w478 -> [w487] mode=indexing
          tunnel: [w486] -> w479 mode=indexing
          tunnel: [w484] -> w476 mode=indexing
          tunnel: w475 -> [w483]
          n210 = Unbundle By Name(w485) -> ("Ch Name"=w488:string)
          n211 = case shown="\"GMU:Source:Release Temp\"" w488 {
            tunnel: w487 -> [_ _ _ _ w511]
            tunnel: [w489 w491 w493 w495 w511] -> w486
            tunnel: w485 -> [w490 w492 w494 w499 w510]
            tunnel: [w490 w492 w494 w498 w510] -> w484
            tunnel: w483 -> [_ _ _ w497 _]
            frame "GMU:Calibration:Gas 1" {
              n212 = local read "Channel 1"() -> (w489:dbl)
            }
            frame "GMU:Calibration:Gas 2" {
              n213 = local read "Channel 2"() -> (w491:dbl)
            }
            frame "GMU:Signal FID:Calib Gas" {
              n214 = local read "Signal FID Calib Gas"() -> (w493:dbl)
            }
            frame "GMU:Source:Release Temp" {
              n215 = local read "Release Temperature"() -> (w496:u16)
              n216 = Equal To 0?(x=w496) -> (x = 0?=w502:bool)
              n217 = case shown="True" w502 {
                tunnel: w496 -> [w504 _]
                tunnel: w497 -> [w507 _]
                tunnel: [w506 ""] -> w500
                tunnel: [w505 w508] -> w501
                frame False {
                  w505 = T3 "Read Ch"  # Module Type
                  n218 = Decrement(x=w504) -> (x-1=w503:u16)
                  n219 = Index Array(array=w507, index=w503) -> (element=w506:string)
                }
                frame True {
                  w508 = T3 "Hold Value"  # Module Type
                }
              }
              n220 = local read "Current Release Temp"() -> (w495:dbl)
              n221 = Bundle By Name(cluster=w499, "String"=w500, "Type"=w501) -> (w498:T2)
            }
            frame "No Match", Default {
            }
          }
        }
      }
      frame "Insert Gas Remaining Info" {
        n222 = local read "Gas Remaining"() -> (w517:string[][])
        n223 = Index Array(array=w517, index (col)=0 ("disabled index (col)")) -> (element=w513:string[])  [unwired: 1 in]
        n224 = for {
          tunnel: w514 -> [w527]
          tunnel: w513 -> [w526] mode=indexing
          tunnel: [w525] -> w512 mode=indexing
          n225 = Concatenate Strings(w527, w526) -> (w525:string)
        }
        n226 = Index Array(array=w517, index (col)=1 ("disabled index (col)")) -> (element=w516:string[])  [unwired: 1 in]
        n227 = for {
          tunnel: w515 -> [w540] mode=indexing
          tunnel: w520 -> [w528] mode=indexing
          tunnel: [w536] -> w521 mode=indexing
          tunnel: w512 -> [w539]
          tunnel: w516 -> [w537]
          n228 = Unbundle By Name(w540) -> ("Ch Name"=w538:string)
          n229 = Search 1D Array(1D array=w539, element=w538) -> (index of element=w534:i32)  [unwired: 1 out]
          n230 = Number To Fractional String(number=w528, precision (6)=i16 3) -> (F-format string=w532:string)  [unwired: 2 out]
          n231 = Index Array(array=w537, index=w534) -> (element=w533:string)
          n232 = Greater Or Equal To 0?(x=w534) -> (x >= 0?=w531:bool)
          n233 = Not Equal?(x=w532, y=w533) -> (x != y?=w530:bool)
          n234 = And(x=w530, y=w531) -> (x .and. y?=w529:bool)
          n235 = case shown="False" w529 {
            tunnel: [w541 w543] -> w536
            tunnel: w533 -> [_ w542]
            tunnel: w528 -> [w541 _]
            frame False {
            }
            frame True {
              n236 = Fract/Exp String To Number(string=w542) -> (number=w543:dbl)  [unwired: 4 out]
            }
          }
        }
      }
      frame "Insert Source info values" {
        n237 = for {
          tunnel: w547 -> [w564] mode=indexing
          tunnel: [w563] -> w555 mode=indexing
          n238 = Unbundle By Name(w564) -> ("Ch Name"=w563:string)
        }
        n239 = Index Array(array="Source Info", index (col)=0 ("disabled index (col)")) -> (element=w551:string[])  [unwired: 1 in]
        n240 = Index Array(array="Source Info", index (col)=1 ("disabled index (col)")) -> (element=w548:string[])  [unwired: 1 in]
        n241 = for {
          tunnel: w555 -> [w562]
          tunnel: w551 -> [w561] mode=indexing
          shift-right: [w558] -> w549
          shift-left: w550 -> [w559]
          tunnel: w548 -> [w557] mode=indexing
          n242 = Fract/Exp String To Number(string=w557) -> (number=w556:dbl)  [unwired: 4 out]
          n243 = Search 1D Array(1D array=w562, element=w561) -> (index of element=w560:i32)  [unwired: 1 out]
          n244 = Replace Array Subset(array=w559, new element=w556, index=w560) -> (w558:dbl[])
        }
      }
      frame "Update Server" {
        w570 = T9 {"Channel Name"="", "New Value"=0.0} ("Update Scan Value Cluster")
        n245 = Index Array(array=w575, index=0 ("Index")) -> (element=w586:T2)
        n246 = local read "Ch Description Array"() -> (w572:T2[])
        n247 = local read "Numerical Values"() -> (w571:dbl[])
        n248 = Initialize Array(w586, 0 ("Dimension Size")) -> (w584:T2[])
        n249 = Initialize Array(w570, 0 ("Dimension Size")) -> (w579:T9[])
        n250 = for {
          shift-right: [w599] -> w581
          shift-left: w584 -> [w600]
          tunnel: w575 -> [w590] mode=indexing
          shift-right: [w598] -> w576
          shift-left: w579 -> [w597]
          tunnel: w574 -> [w592] mode=indexing
          tunnel: w572 -> [w591] mode=indexing
          tunnel: w571 -> [w595] mode=indexing
          tunnel: w570 -> [w593]
          n251 = Equal?(x=w590, y=w591) -> (x = y?=w596:bool)
          n252 = Equal?(x=w592, y=w595) -> (x = y?=w594:bool)
          n253 = case shown="False" w594 {
            tunnel: w597 -> [w607 w608]
            tunnel: [w606 w608] -> w598
            tunnel: w593 -> [w605 _]
            tunnel: w592 -> [w604 _]
            tunnel: w590 -> [w603 _]
            frame False {
              n254 = Unbundle By Name(w603) -> ("Ch Name"=w602:string)
              n255 = Bundle By Name(cluster=w605, "Channel Name"=w602, "New Value"=w604) -> (w601:T9)
              n256 = Build Array (concatenate)(w607, w601) -> (w606:T9[])
            }
            frame True {
            }
          }
          n257 = case shown="False" w596 {
            tunnel: w600 -> [w611 w612]
            tunnel: w590 -> [w610 _]
            tunnel: [w609 w612] -> w599
            frame False {
              n258 = Build Array (concatenate)(w611, w610) -> (w609:T2[])
            }
            frame True {
            }
          }
        }
        n259 = Array Size(array=w581) -> (size(s)=w583:i32)
        n260 = Array Size(array=w576) -> (size(s)=w577:i32)
        n261 = Greater Than 0?(x=w583) -> (x > 0?=w582:bool)
        n262 = Greater Than 0?(x=w577) -> (x > 0?=w578:bool)
        n263 = case shown="True" w582 {
          tunnel: w581 -> [_ w589]
          frame False {
          }
          frame True {
            n264 = call "Update_Ch_Discription_client.vi"("Channels to update In"=w589) -> ()  [unwired: 1 out]
          }
        }
        n265 = case shown="True" w578 {
          tunnel: w576 -> [_ w588]
          frame False {
          }
          frame True {
            n266 = call "Update_Current_Value_client.vi"("Update array in"=w588) -> ()  [unwired: 1 in]
          }
        }
        n267 = Select(t="Select Server Channels", s="Select Plug Ins", f="Close Panel") -> (s? t:f=w566:string)
      }
      frame "Select Server Channels" {
        w616 = string[] []
        w625 = T10."Zero or more"  # Selector mode
        n268 = local read "Source Info"() -> (w623:string[][])
        n269 = global read "Preference_global.vi" "Rig Setup"() -> (w636:string)
        n270 = Concatenate Strings(w636, ":" ("string")) -> (w633:string)
        n271 = String Length(string=w633) -> (length=w634:i32)
        n272 = call "Get_ADAM_Ch_names_client.vi"("Channel names set"=Channel_names."All Channels") -> ("Ch names"=w626:string[])
        n273 = Index Array(array=w623, index (col)=0) -> (element=w618:string[])  [unwired: 1 in]
        n274 = for {
          tunnel: w634 -> [w669]
          tunnel: w626 -> [w659] mode=indexing
          tunnel: w633 -> [w661]
          shift-right: [w663] -> w624
          shift-left: string[] [] -> [w664]
          n275 = Search/Split String(string=w659, offset (0)=w669) -> (substring before match=w668:string, match + rest of string=w667:string)  [unwired: 2 out]
          n276 = Equal?(x=w661, y=w668) -> (x = y?=w657:bool)
          n277 = Match Pattern(string=w667, regular expression="[Ss]ource") -> (offset past match=w665:i32)  [unwired: 4 out]
          n278 = Concatenate Strings(w661, "Source:Status") -> (w660:string)
          n279 = Greater Or Equal To 0?(x=w665) -> (x >= 0?=w658:bool)
          n280 = Equal?(x=w660, y=w659) -> (x = y?=w656:bool)
          n281 = Compound Arithmetic op=AND(invert w656, w657, w658) -> (w655:bool)
          n282 = case shown="True" w655 {
            tunnel: w664 -> [w670 w673]
            tunnel: w659 -> [_ w671]
            tunnel: [w670 w672] -> w663
            frame False {
            }
            frame True {
              n283 = Build Array (concatenate)(w673, w671) -> (w672:string[])
            }
          }
        }
        n284 = call "Select_Strings.vi"("Available Ch names"=w624, "Message"="Please select the appropriate source information channels", "Selector mode"=w625, "Desired Ch names (in)"=w618) -> ("Selected Channel Names"=w617:string[])  [unwired: 4 out]
        n285 = for {
          tunnel: w618 -> [w640] mode=indexing
          tunnel: w617 -> [w641]
          shift-right: [w637] -> w615
          shift-left: w616 -> [w638]
          n286 = Search 1D Array(1D array=w641, element=w640) -> (index of element=w639:i32)  [unwired: 1 out]
          n287 = case shown="-1" w639 {
            tunnel: w640 -> [_ w645]
            tunnel: w638 -> [w642 w644]
            tunnel: [w642 w643] -> w637
            frame 0, Default {
            }
            frame -1 {
              n288 = Build Array (concatenate)(w644, w645) -> (w643:string[])
            }
          }
        }
        n289 = call "Adam_Ch_on_off.vi"("Ch State"=Channel_State."Always Off", "ADAM Ch Names"=w615) -> ()  [unwired: 1 out]
        n290 = for {
          tunnel: w617 -> [w649] mode=indexing
          tunnel: w618 -> [w650]
          shift-right: [w646] -> w619
          shift-left: w616 -> [w647]
          n291 = Search 1D Array(1D array=w650, element=w649) -> (index of element=w648:i32)  [unwired: 1 out]
          n292 = case shown="-1" w648 {
            tunnel: w649 -> [_ w654]
            tunnel: w647 -> [w651 w653]
            tunnel: [w651 w652] -> w646
            frame 0, Default {
            }
            frame -1 {
              n293 = Build Array (concatenate)(w653, w654) -> (w652:string[])
            }
          }
        }
        n294 = call "Adam_Ch_on_off.vi"("Ch State"=Channel_State."On", "ADAM Ch Names"=w619) -> ()  [unwired: 1 out]
      }
      frame "Close Panel" {
        n295 = local read "dup reference"() -> (w675:refnum<vi>)
        n296 = property class="VI"(reference=w675, "Front Panel Window:Open"=FALSE) -> (reference out=w677:refnum<vi>, error out=w676:errorcluster)  [unwired: 1 in]
        n297 = Close Reference(reference=w677, error in (no error)=w676) -> ()  [unwired: 1 out]
      }
    }
  }
